vi "pick 1 ball.vi"   [LabVIEW 2016, in "Test2.lvrbt"]
uses:
  Test2.lvrbt
  <vilib>/NXT/Block Support/NXT_InputPort.ctl
  <vilib>/NXT/Hardware/Plugins/Tetrix DC Motor/TetrixDCMotorAddress.ctl
  <vilib>/NXT/Hardware/Plugins/Tetrix 180 deg Servo/Tetrix180ServoAddress.ctl
  <vilib>/NXT/NXTIO Xnodes/NXTIONodeSubVIs/TETRIX IO Move Servos.vi
  <vilib>/NXT/Dual Mode Library/Waits/Wait_Num.vi
  <vilib>/NXT/NXTIO Xnodes/NXTIONodeSubVIs/TETRIX IO Move DC Motors.vi
  <vilib>/NXT/Dual Mode Library/Waits/Wait_EV3_Ultrasonic_Centimeters_Further.vi
  <vilib>/NXT/NXTIO Xnodes/NXTIONodeSubVIs/TETRIX IO Stop DC Motors.vi
  <vilib>/NXT/Dual Mode Library/Waits/Wait_EV3_Ultrasonic_Centimeter_Closer.vi
  <vilib>/NXT/NXTIO Xnodes/AddressXNode/NXTIOAddress.xnode
  <vilib>/NXT/Subs/LVHSConnector.ctl
  <vilib>/NXT/NXTIO Xnodes/NXTIOXNode/NXTIO.xnode
  <vilib>/NXT/LegoClasses/BrickReference/BrickReference.lvclass
types:
  T1 = typedef "NXT_InputPort.ctl" = u32
  T2 = typedef "Tetrix180ServoAddress.ctl" = i32
  T3 = cluster{"Tetrix180Servo":T2, "Tetrix180Servo":T2, "Tetrix180Servo":T2, "Tetrix180Servo":T2, "Tetrix180Servo":T2, "Tetrix180Servo":T2}
  T4 = typedef "LVHSConnector.ctl" = refnum<class "BrickReference.lvclass">
  T5 = typedef "TetrixDCMotorAddress.ctl" = i32
  T6 = cluster{"TetrixDCMotor":T5, "TetrixDCMotor 2":T5}
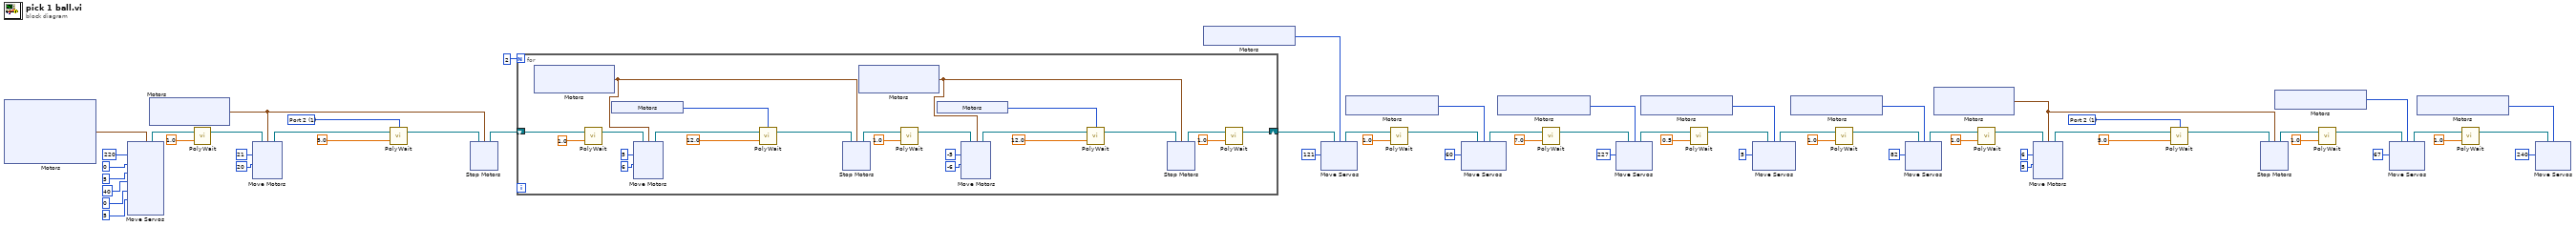
[diagram p0: block diagram]
diagram:
  w11 = T1 1 items=["Port 1", "Port 2", "Port 3", "Port 4"] ("Port (Port 1)")
  w59 = T1 1 items=["Port 1", "Port 2", "Port 3", "Port 4"] ("Port (Port 1)")
  n1 = xnode "Motors"() -> ("Motor"=w42:T3)
  n2 = xnode "Move Servos"("Position 6"=u8 5, "Position 5"=u8 0, "Position 4"=u8 40, "Position 3"=u8 5, "Position 2"=u8 0, "Position 1"=u8 220, "Motors"=w42) -> ("NXT/EV3"=w9:T4)  [unwired: 1 in]
  n3 = xnode "Motors"() -> ("Motor"=w12:cluster{"TetrixDCMotor":T5, "TetrixDCMotor":T5})
  n4 = call-poly <vilib>:"PolyWait.vi"("Time (1 sec)"=sgl 1.0, "NXT/EV3"=w9) -> ("NXT/EV3"=w8:T4)  [unwired: 2 in]
  n5 = xnode "Move Motors"("Power/Speed 2"=i8 20, "Power/Speed 1"=i8 21, "Motors"=w12, "NXT/EV3"=w8) -> ("NXT/EV3"=w15:T4)
  n6 = call-poly <vilib>:"PolyWait.vi"("Centimeters (50)"=sgl 5.0, "NXT/EV3"=w15, "Port (Port 1)"=w11) -> ("NXT/EV3"=w13:T4)  [unwired: 1 in]
  n7 = xnode "Stop Motors"("Motors"=w12, "NXT/EV3"=w13) -> ("NXT/EV3"=w2:T4)
  n8 = for {
    N: 2 -> [_]
    shift-right: [w64] -> w1
    shift-left: w2 -> [w63]
    n9 = xnode "Motors"() -> ("Motor"=w78:cluster{"TetrixDCMotor":T5, "TetrixDCMotor":T5})
    n10 = call-poly <vilib>:"PolyWait.vi"("Time (1 sec)"=sgl 1.0, "NXT/EV3"=w63) -> ("NXT/EV3"=w77:T4)  [unwired: 2 in]
    n11 = xnode "Motors"() -> ("Sensor"=w80:T1)
    n12 = xnode "Move Motors"("Power/Speed 2"=i8 6, "Power/Speed 1"=i8 5, "Motors"=w78, "NXT/EV3"=w77) -> ("NXT/EV3"=w82:T4)
    n13 = call-poly <vilib>:"PolyWait.vi"("Centimeters (40)"=sgl 12.0, "NXT/EV3"=w82, "Port (Port 1)"=w80) -> ("NXT/EV3"=w79:T4)  [unwired: 1 in]
    n14 = xnode "Stop Motors"("Motors"=w78, "NXT/EV3"=w79) -> ("NXT/EV3"=w76:T4)
    n15 = xnode "Motors"() -> ("Motor"=w69:cluster{"TetrixDCMotor":T5, "TetrixDCMotor":T5})
    n16 = call-poly <vilib>:"PolyWait.vi"("Time (1 sec)"=sgl 1.0, "NXT/EV3"=w76) -> ("NXT/EV3"=w72:T4)  [unwired: 2 in]
    n17 = xnode "Motors"() -> ("Sensor"=w67:T1)
    n18 = xnode "Move Motors"("Power/Speed 2"=i8 -6, "Power/Speed 1"=i8 -5, "Motors"=w69, "NXT/EV3"=w72) -> ("NXT/EV3"=w71:T4)
    n19 = call-poly <vilib>:"PolyWait.vi"("Centimeters (50)"=sgl 12.0, "NXT/EV3"=w71, "Port (Port 1)"=w67) -> ("NXT/EV3"=w70:T4)  [unwired: 1 in]
    n20 = xnode "Stop Motors"("Motors"=w69, "NXT/EV3"=w70) -> ("NXT/EV3"=w65:T4)
    n21 = call-poly <vilib>:"PolyWait.vi"("Time (1 sec)"=sgl 1.0, "NXT/EV3"=w65) -> ("NXT/EV3"=w64:T4)  [unwired: 2 in]
  }
  n22 = xnode "Motors"() -> ("Motor"=w7:T2)
  n23 = xnode "Move Servos"("Position 1"=u8 121, "Motors"=w7, "NXT/EV3"=w1) -> ("NXT/EV3"=w5:T4)
  n24 = xnode "Motors"() -> ("Motor"=w54:T2)
  n25 = call-poly <vilib>:"PolyWait.vi"("Time (1 sec)"=sgl 1.0, "NXT/EV3"=w5) -> ("NXT/EV3"=w29:T4)  [unwired: 2 in]
  n26 = xnode "Move Servos"("Position 1"=u8 60, "Motors"=w54, "NXT/EV3"=w29) -> ("NXT/EV3"=w51:T4)
  n27 = xnode "Motors"() -> ("Motor"=w50:T2)
  n28 = call-poly <vilib>:"PolyWait.vi"("Time (1 sec)"=sgl 7.0, "NXT/EV3"=w51) -> ("NXT/EV3"=w48:T4)  [unwired: 2 in]
  n29 = xnode "Move Servos"("Position 1"=u8 227, "Motors"=w50, "NXT/EV3"=w48) -> ("NXT/EV3"=w46:T4)
  n30 = xnode "Motors"() -> ("Motor"=w45:T2)
  n31 = call-poly <vilib>:"PolyWait.vi"("Time (1 sec)"=sgl 0.5, "NXT/EV3"=w46) -> ("NXT/EV3"=w43:T4)  [unwired: 2 in]
  n32 = xnode "Move Servos"("Position 1"=u8 5, "Motors"=w45, "NXT/EV3"=w43) -> ("NXT/EV3"=w35:T4)
  n33 = xnode "Motors"() -> ("Motor"=w33:T2)
  n34 = call-poly <vilib>:"PolyWait.vi"("Time (1 sec)"=sgl 1.0, "NXT/EV3"=w35) -> ("NXT/EV3"=w32:T4)  [unwired: 2 in]
  n35 = xnode "Move Servos"("Position 1"=u8 82, "Motors"=w33, "NXT/EV3"=w32) -> ("NXT/EV3"=w31:T4)
  n36 = xnode "Motors"() -> ("Motor"=w57:cluster{"TetrixDCMotor":T5, "TetrixDCMotor":T5})
  n37 = call-poly <vilib>:"PolyWait.vi"("Time (1 sec)"=sgl 1.0, "NXT/EV3"=w31) -> ("NXT/EV3"=w55:T4)  [unwired: 2 in]
  n38 = xnode "Move Motors"("Power/Speed 2"=i8 5, "Power/Speed 1"=i8 6, "Motors"=w57, "NXT/EV3"=w55) -> ("NXT/EV3"=w60:T4)
  n39 = call-poly <vilib>:"PolyWait.vi"("Centimeters (50)"=sgl 5.0, "NXT/EV3"=w60, "Port (Port 1)"=w59) -> ("NXT/EV3"=w58:T4)  [unwired: 1 in]
  n40 = xnode "Stop Motors"("Motors"=w57, "NXT/EV3"=w58) -> ("NXT/EV3"=w26:T4)
  n41 = xnode "Motors"() -> ("Motor"=w24:T2)
  n42 = call-poly <vilib>:"PolyWait.vi"("Time (1 sec)"=sgl 1.0, "NXT/EV3"=w26) -> ("NXT/EV3"=w23:T4)  [unwired: 2 in]
  n43 = xnode "Move Servos"("Position 1"=u8 67, "Motors"=w24, "NXT/EV3"=w23) -> ("NXT/EV3"=w21:T4)
  n44 = xnode "Motors"() -> ("Motor"=w19:T2)
  n45 = call-poly <vilib>:"PolyWait.vi"("Time (1 sec)"=sgl 1.0, "NXT/EV3"=w21) -> ("NXT/EV3"=w18:T4)  [unwired: 2 in]
  n46 = xnode "Move Servos"("Position 1"=u8 240, "Motors"=w19, "NXT/EV3"=w18) -> ()  [unwired: 1 out]
